vi "PulseTrain (G3)-Compute Max Level.vi"(0 "Pulse Train Params":T4, 5 "Filter":T3 {"IIR Filter Cluster"."Forward Coefficients" format="%.4f"; "IIR Filter Cluster"."Reverse Coefficients" format="%.4f"}, 9 "Level":T1, 11 "error in (no error)":errorcluster, 12 "Sampling Rate (Hz)":dbl, 13 "Npts":i32) -> (6 "Max Level":dbl, 10 "Level out":T1, 15 "error out":errorcluster)   [LabVIEW 2020]
uses:
  Waveform VIs/Pulse Train VIs/Pulse Train Params.ctl
  Waveform VIs/Pulse Train VIs/Pulse Polarity.ctl
  Waveform VIs/Pulse Train VIs/PT-Continuous State.ctl
  Controls/Filter XCtl/Filter Data.ctl
  XControls/Level (G3)/Level Data.ctl
  XControls/Level (G3)/Level Units (G3).ctl
  <vilib>/Analysis/2dsp.llb/Inverse Complex FFT.vi
  PXI DAQ VIs/DAQ Engine VIs/PXI Globals.vi
  Utility VIs/Math VIs/Linear to dB (scalar).vi
  <vilib>/Analysis/NI_AALPro.lvlib
  Controls/Filter XCtl/Filter XCtl.xctl
  XControls/Level (G3)/Level (G3).xctl
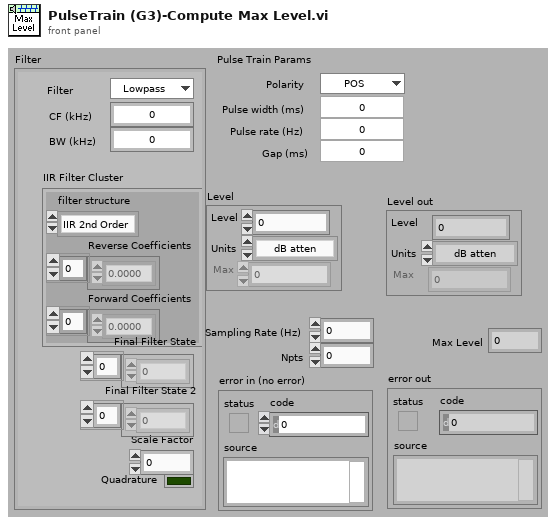
[diagram p1: front panel]
types:
  T1 = typedef "Level (G3).xctl/Level Data.ctl" = cluster{"Level":dbl, "Units":T2, "Max":dbl, "Data":cluster{"Multiplier":dbl, "Cal File":path, "Cal":cluster{"Freq (Hz)":dbl[], "Mag (dB SPL)":dbl[], "Phase (deg)":dbl[]}, "audiogram":path}}
  T2 = typedef "Level (G3).xctl/Level Units (G3).ctl" = enum16{"dB atten", "dB SPL", "dB re 1 Vrms", "dB V/Hz½", "mW", "dB HL", "Volts", "dB mW"}
  T3 = typedef "Filter XCtl.xctl/Filter Data.ctl" = cluster{"CF (kHz)":dbl, "BW (kHz)":dbl, "IIR Filter Cluster":cluster{"filter structure":enum32{"IIR 2nd Order", "IIR 4th Order"}, "Reverse Coefficients":dbl[], "Forward Coefficients":dbl[]}, "Final Filter State":dbl[], "Scale Factor":dbl, "Final Filter State 2":dbl[], "Quadrature":bool, "Type":enum16{"Lowpass", "Highpass", "Bandpass", "Bandstop", "OFF"}}
  T4 = typedef "Pulse Train Params.ctl" = cluster{"Pulse width (us)":dbl, "Pulse rate (Hz)":dbl, "Gap (ms)":dbl, "Polarity":T5, "PT State":T6, "Asynch":bool}
  T5 = typedef "Pulse Polarity.ctl" = enum16{"POS", "NEG", "POS-NEG", "NEG-POS"}
  T6 = typedef "PT-Continuous State.ctl" = cluster{"Template":dbl[], "Nperiod":i32, "Index":i32, "Pulse Rate (Hz)":dbl, "Phase (cycles)":dbl, "Noff":i32}
  T7 = typedef "LaserCal-Data (PT).ctl" = cluster{"I-O":cluster{"Volts":dbl[], "Width":dbl[], "Rate":dbl[], "Power":dbl[][][][]}, "Data header":string, "Tsettle (s)":dbl}
  T8 = cluster{"Volts":dbl[], "Width":dbl[], "Rate":dbl[], "Power":dbl[][][][]}
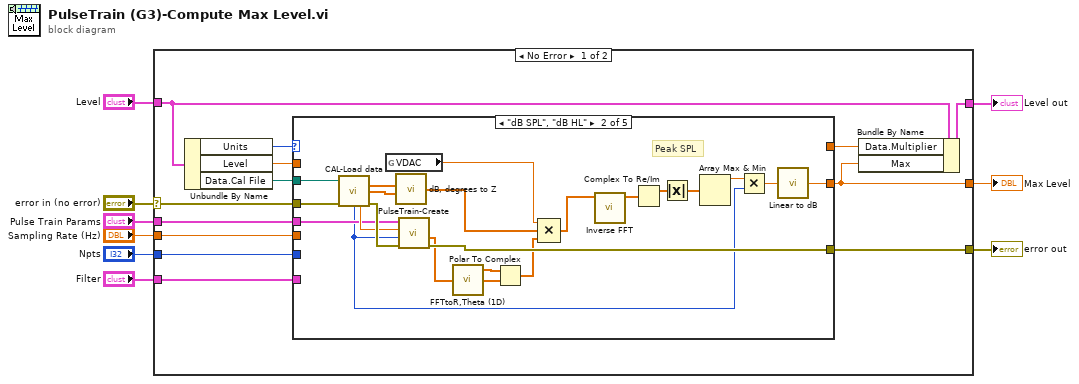
[diagram p0: block diagram]
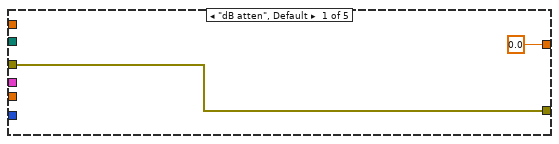
[diagram p2: hidden frame]
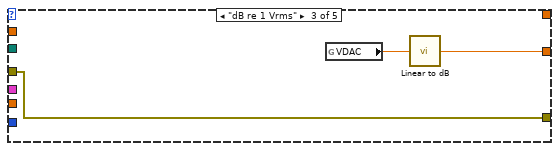
[diagram p3: hidden frame]
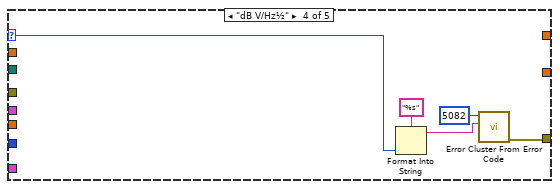
[diagram p4: hidden frame]
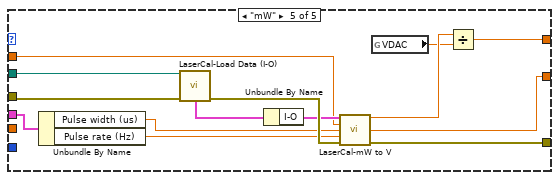
[diagram p5: hidden frame]
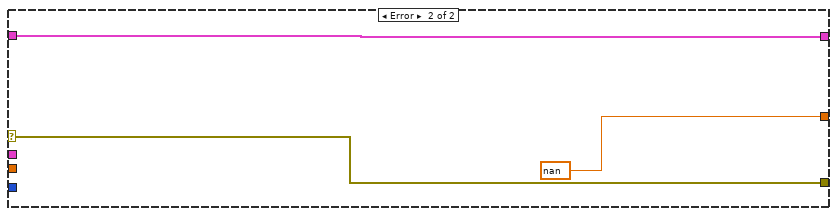
[diagram p6: hidden frame]
diagram:
  n1 = case shown="No Error" "error in (no error)" {
    selector: "error in (no error)" -> [w22 w71]
    tunnel: "Level" -> [w17 w69]
    tunnel: "Pulse Train Params" -> [w12 _]
    tunnel: "Filter" -> [w20 _]
    tunnel: [w18 w71] -> w8
    tunnel: "Npts" -> [w21 _]
    tunnel: [w16 nan ("Reference Level")] -> w3
    tunnel: "Sampling Rate (Hz)" -> [w19 _]
    tunnel: [w15 w69] -> w1
    frame No Error {
      n2 = Unbundle By Name(w17) -> ("Units"=w14:T2, "Level"=w10:dbl, "Data.Cal File"=w13:path)
      n3 = case shown="\"dB SPL\", \"dB HL\"" w14 {
        selector: w14 -> [_ _ _ w50 _]
        tunnel: w22 -> [w23 w46 w47 _ w68]
        tunnel: w21 -> [_ _ _ _ _]
        tunnel: w20 -> [_ _ _ _ _]
        tunnel: [0.0 ("Reference Level") w25 w48 _ w60] -> w16
        tunnel: w19 -> [_ _ _ _ _]
        tunnel: [w23 w39 w47 w51 w65] -> w18
        tunnel: w13 -> [_ w45 _ _ w56]
        tunnel: w12 -> [_ w38 _ _ w67]
        tunnel: [_ _ _ _ w57] -> w11
        tunnel: w10 -> [_ _ _ _ w55]
        frame "dB atten", Default {
        }
        frame "dB SPL", "dB HL" {
          # "Peak SPL"
          n4 = call "CAL-Load data.vi"("user path"=w45, "error in (no error)"=w46) -> ("Mag"=w44:dbl[], "Phase"=w43:dbl[], "npts"=w27:i32, "Fs (Hz)"=w40:dbl, "error out"=w41:errorcluster)  [unwired: 6 in, 3 out]
          n5 = global read "PXI Globals.vi" "VDAC"() -> (w37:dbl)
          n6 = call "dB, degrees to Z.vi"("Magnitude (dB)"=w44, "Phase (degrees)"=w43) -> ("Z"=w42:cdb[])  [unwired: 5 in]
          n7 = call "PulseTrain-Create.vi"("error in (no error)"=w41, "Npts"=w27, "Sampling Rate (Hz)"=w40, "Pulse Train Params"=w38) -> ("error out"=w39:errorcluster, "Waveform"=w36:dbl[])  [unwired: 4 in, 2 out]
          n8 = call "FFTtoR,Theta (1D).VI"("X"=w36) -> ("+Freq. Mag of FFT"=w34:dbl[], "+Freq Theta of FFT"=w35:dbl[])  [unwired: 1 in]
          n9 = Polar To Complex(1:w35, 2:w34) -> (0:w33:cdb[])
          n10 = Compound Arithmetic op=MULTIPLY(w37, w42, w33) -> (w32:cdb[])
          n11 = call-poly <vilib>:"Inverse FFT.vi"("FFT {X}"=w32) -> ("X"=w31:cdb[])  [unwired: 9 in, 1 out]
          n12 = Complex To Re/Im(x + iy=w31) -> (x=w30:dbl[])  [unwired: 1 out]
          n13 = Absolute Value(x=w30) -> (abs(x)=w28:dbl[])
          n14 = Array Max & Min(array=w28) -> (max value=w29:dbl)  [unwired: 3 out]
          n15 = Multiply(x=w29, y=w27) -> (x*y=w26:dbl)
          n16 = call-poly "Linear to dB.vi"("Linear"=w26) -> ("dB"=w25:dbl)
        }
        frame "dB re 1 Vrms" {
          n17 = global read "PXI Globals.vi" "VDAC"() -> (w49:dbl)
          n18 = call-poly "Linear to dB.vi"("Linear"=w49) -> ("dB"=w48:dbl)
        }
        frame "dB V/Hz½" {
          n19 = Format Into String(format string="%s", w50) -> (resulting string=w53:string)  [unwired: 2 in, 1 out]
          n20 = call <vilib>:"Error Cluster From Error Code.vi"("error message (\"\")"=w53, "error code (0)"=5082) -> ("error out"=w51:errorcluster)  [unwired: 7 in]
        }
        frame "mW" {
          n21 = Unbundle By Name(w67) -> ("Pulse width (us)"=w61:dbl, "Pulse rate (Hz)"=w64:dbl)
          n22 = call "LaserCal-Load Data (I-O).vi"("Path"=w56, "error in (no error)"=w68) -> ("I-O Data"=w63:T7, "error out"=w66:errorcluster)  [unwired: 6 in, 6 out]
          n23 = Unbundle By Name(w63) -> ("I-O"=w62:T8)
          n24 = call "LaserCal-mW to V.vi"("I-O"=w62, "Power (mW)"=w55, "Pulse width (us)"=w61, "Pulse rate (Hz)"=w64, "error in (no error)"=w66) -> ("Volts"=w59:dbl, "Max (mW)"=w60:dbl, "error out"=w65:errorcluster)  [unwired: 8 in]
          n25 = global read "PXI Globals.vi" "VDAC"() -> (w58:dbl)
          n26 = Divide(x=w59, y=w58) -> (x/y=w57:dbl)
        }
      }
      n27 = Bundle By Name(cluster=w17, "Data.Multiplier"=w11, "Max"=w16) -> (w15:T1)
    }
    frame Error {
    }
  }
  "error out" <- w8
  "Max Level" <- w3
  "Level out" <- w1
